vi "SplitControlPath.vi"(8 "error in":errorcluster, 11 "control path string":string) -> (0 "error out":errorcluster, 3 "string array":string[](array[string]))   [LabVIEW 2021]
uses:
  <vilib>/regexp/Match Regular Expression.xnode
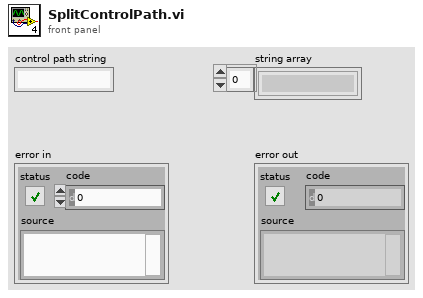
[diagram p1: front panel]
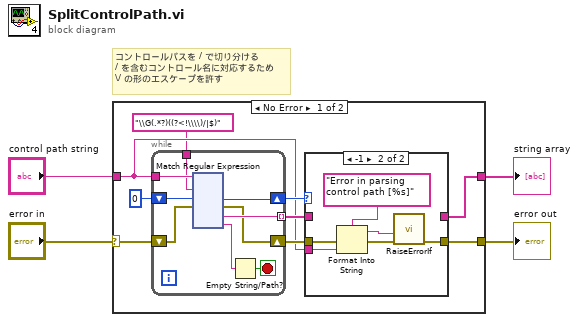
[diagram p0: block diagram]
diagram:
  # "コントロールパスを / で切り分ける\n/ を含むコントロール名に対応するため\n\\/ の形のエスケープを許す"
  n1 = case shown="No Error" "error in" {
    selector: "error in" -> [w6 w151]
    tunnel: [w9 _] -> w4
    tunnel: [w8 w151] -> w3
    tunnel: "control path string" -> [w7 _]
    frame No Error {
      n2 = while {
        shift-right: [w21] -> w11
        shift-left: 0 -> [w22]
        shift-right: [w15] -> w12
        shift-left: w6 -> [w20]
        tunnel: w7 -> [w19]
        tunnel: [w16] -> w10 mode=indexing
        tunnel: "\\G(.*?)((?<!\\\\)/|$)" -> [w14]
        stop <- w18 stop-if-true
        n3 = xnode "Match Regular Expression"("input string"=w19, "regular expression"=w14, "offset (0)"=w22, "error in"=w20) -> ("offset past match"=w21:i32, "error out"=w15:errorcluster, "submatch 1"=w16:string, "submatch 2"=w17:string)  [unwired: 2 in, 3 out]
        n4 = Empty String/Path?(string/path=w17) -> (empty?=w18:bool)
      }
      n5 = case shown="-1" w11 {
        tunnel: w12 -> [w143 w147]
        tunnel: w10 -> [w144 _]
        tunnel: [w144 _] -> w9
        tunnel: [w143 w150] -> w8
        tunnel: w7 -> [_ w149]
        frame Default {
        }
        frame -1 {
          n6 = Format Into String(format string="Error in parsing control path [%s]", error in=w147, w149) -> (resulting string=w148:string, error out=w146:errorcluster)  [unwired: 1 in]
          n7 = call "RaiseErrorIf.vi"("error in (no error)"=w146, "error message"=w148) -> ("error out"=w150:errorcluster)  [unwired: 9 in]
        }
      }
    }
    frame Error {
    }
  }
  "string array" <- w4
  "error out" <- w3
